vi "Feedback Picture.vi"(5 "Unused":bool, 7 "Open State":T3, 10 "Closed State":T3, 11 "Feedback Pictures":T2) -> (2 "Feedback Picture":T1)   [LabVIEW 2023, in "VolatusGUIElements.lvlib" / "2WayValveV.lvclass"]
uses:
  2WayValveV.lvclass
  Channel State.ctl
  Feedback Pictures.ctl
  2WayValveV.lvclass/2WayValveV.ctl
  Picture.ctl
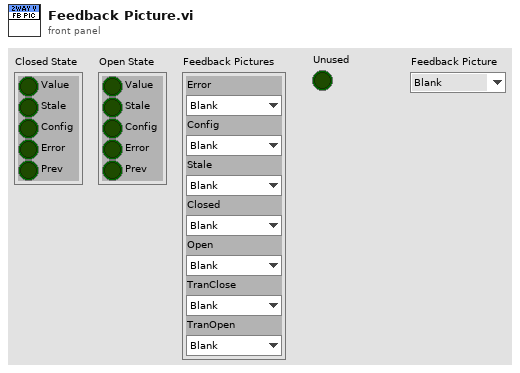
[diagram p1: front panel]
types:
  T1 = typedef "VolatusGUIElements.lvlib/2WayValveV.lvclass/Picture.ctl" = enum16{"Blank", "OutClose", "OutOpen", "OutTranClose", "OutTranOpen", "OutConfig", "OutStale", "OutError", "InClose", "InOpen", "InTranClose", "InTranOpen", "InConfig", "InStale", "InError", "EnOff", "EnOn", "EnConfig", "EnStale", "EnError"}
  T2 = typedef "VolatusGUIElements.lvlib/2WayValveV.lvclass/Feedback Pictures.ctl" = cluster{"Error":T1, "Config":T1, "Stale":T1, "Closed":T1, "Open":T1, "TranClose":T1, "TranOpen":T1}
  T3 = typedef "VolatusGUIElements.lvlib/2WayValveV.lvclass/Channel State.ctl" = cluster{"Value":bool, "Stale":bool, "Config":bool, "Error":bool, "Prev":bool}
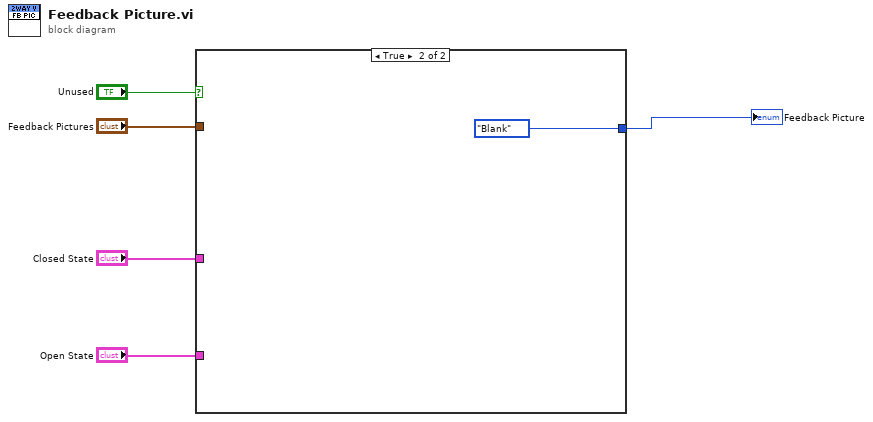
[diagram p0: block diagram]
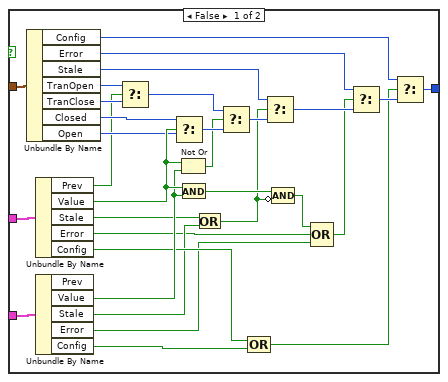
[diagram p2: hidden frame]
diagram:
  n1 = case shown="True" "Unused" {
    tunnel: "Feedback Pictures" -> [w36 _]
    tunnel: "Closed State" -> [w35 _]
    tunnel: "Open State" -> [w34 _]
    tunnel: [w16 Picture."Blank" ("Open")] -> w1
    frame False {
      n2 = Unbundle By Name(w36) -> ("Config"=w18:T1, "Error"=w22:T1, "Stale"=w24:T1, "TranOpen"=w15:T1, "TranClose"=w14:T1, "Closed"=w13:T1, "Open"=w12:T1)
      n3 = Unbundle By Name(w35) -> ("Prev"=w11:bool, "Value"=w31:bool, "Stale"=w26:bool, "Error"=w21:bool, "Config"=w28:bool)
      n4 = Unbundle By Name(w34) -> ("Value"=w30:bool, "Stale"=w25:bool, "Error"=w20:bool, "Config"=w29:bool)  [unwired: 1 out]
      n5 = Select(t=w15, s=w11, f=w14) -> (s? t:f=w10:T1)
      n6 = Select(t=w13, s=w31, f=w12) -> (s? t:f=w33:T1)
      n7 = Not Or(1:w30, 2:w31) -> (0:w32:bool)
      n8 = And(x=w31, y=w30) -> (x .and. y?=w9:bool)
      n9 = Or(x=w26, y=w25) -> (x .or. y?=w6:bool)
      n10 = Select(t=w10, s=w32, f=w33) -> (s? t:f=w27:T1)
      n11 = Compound Arithmetic op=OR(w28, w29) -> (w17:bool)
      n12 = Select(t=w24, s=w6, f=w27) -> (s? t:f=w23:T1)
      n13 = Compound Arithmetic op=AND(w9, invert w6) -> (w8:bool)
      n14 = Compound Arithmetic op=OR(w8, w21, w20) -> (w7:bool)
      n15 = Select(t=w22, s=w7, f=w23) -> (s? t:f=w19:T1)
      n16 = Select(t=w18, s=w17, f=w19) -> (s? t:f=w16:T1)
    }
    frame True {
    }
  }
  "Feedback Picture" <- w1
